vi "Get Full Help.vi"(8 "error in (no error)":errorcluster, 11 "Help in":refnum<class "Help.lvclass">) -> (0 "error out":errorcluster, 2 "Full Help":string, 3 "Help out":refnum<class "Help.lvclass">)   [LabVIEW 2020, in "Help.lvlib" / "Help.lvclass"]
uses:
  Help.lvclass
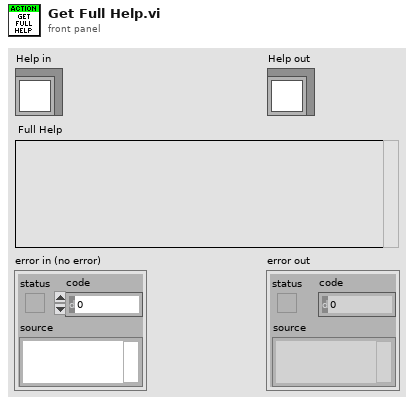
[diagram p1: front panel]
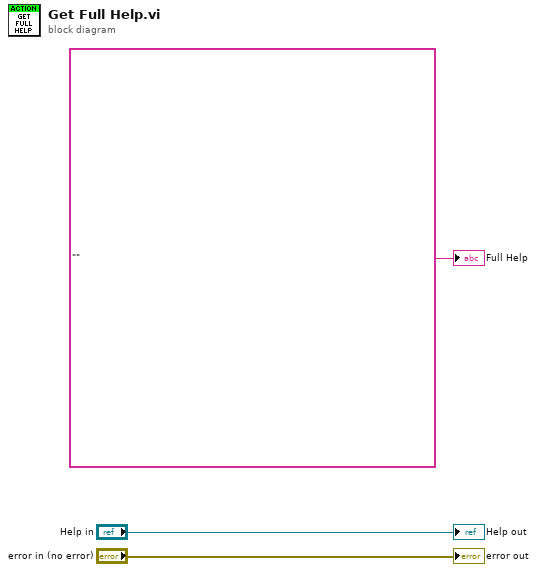
[diagram p0: block diagram]
diagram:
  "error out" <- "error in (no error)"
  "Help out" <- "Help in"
  "Full Help" <- "" ("Full Help")
